vi "字符串匹配测试.vi"() -> ()   [LabVIEW 2019, in "test.lvlib"]
uses:
  SubVI/test.lvlib
panel:
  out "匹配后偏移量":i32
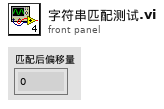
[diagram p1: front panel]
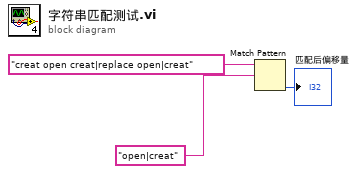
[diagram p0: block diagram]
diagram:
  n1 = Match Pattern(string="creat open creat|replace open|creat" ("字符串"), regular expression="open|creat" ("正则表达式")) -> (offset past match=→"匹配后偏移量":i32)  [unwired: 1 in, 3 out]
